vi "Mediaplayer mute.vi"(8 "error in (no error)":errorcluster, 10 "mute":bool, 11 "Refnum":refnum<k7>) -> (0 "error out":errorcluster)   [LabVIEW 2010]
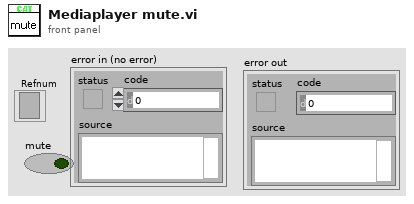
[diagram p1: front panel]
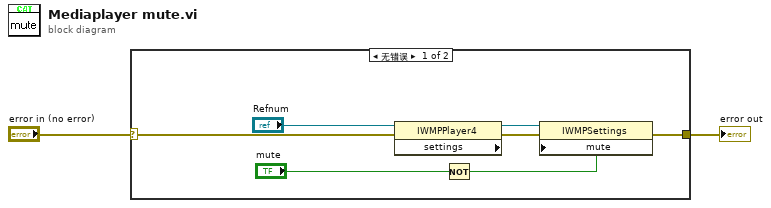
[diagram p0: block diagram]
diagram:
  n1 = case shown="无错误" "error in (no error)" {
    selector: "error in (no error)" -> [w5 w10]
    tunnel: [w4 w10] -> w1
    frame No Error {
      n2 = property class="IWMPPlayer4"(reference="Refnum", error in=w5) -> (error out=w6:errorcluster, "settings"=w8:refnum<k7>)  [unwired: 1 out]
      n3 = Not(x="mute") -> (.not. x?=w3:bool)
      n4 = property class="IWMPSettings"(reference=w8, error in=w6, "mute"=w3) -> (error out=w4:errorcluster)  [unwired: 1 out]
    }
    frame Error {
    }
  }
  "error out" <- w1
